vi "ParseArrayOfVariants.vi"(2 "Types":variant[](array[variant]), 6 "Type":enum16{"Indicators", "Controls"}(ring)) -> (15 "Funcdefinition":string, 16 "Description":string, 17 "FuncString":string)   [LabVIEW 2018, in "Matlab.lvclass"]
uses:
  Matlab.lvclass
  <vilib>/Utility/Data Type/NI_Data Type.lvlib
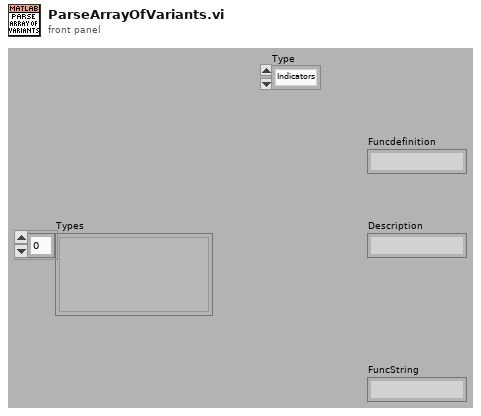
[diagram p1: front panel]
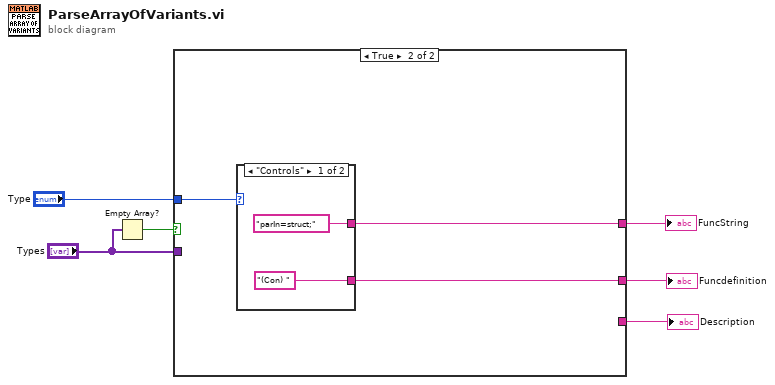
[diagram p0: block diagram]
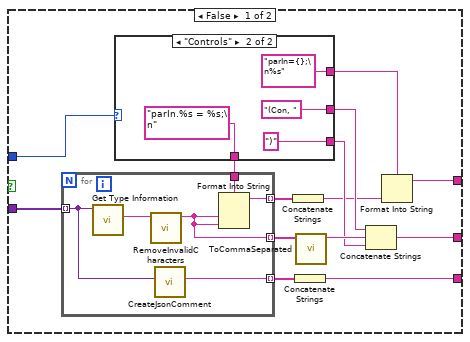
[diagram p2: hidden frame]
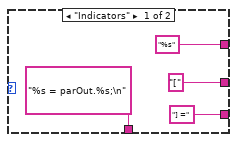
[diagram p3: hidden frame]
diagram:
  n1 = Empty Array?(array="Types") -> (empty?=w1:bool)
  n2 = case shown="True" w1 {
    tunnel: [w14 w37] -> w3
    tunnel: [w18 _] -> w2
    tunnel: [w7 w35] -> w4
    tunnel: "Types" -> [w15 _]
    tunnel: "Type" -> [w13 w36]
    frame False {
      n3 = case shown="\"Controls\"" w13 {
        tunnel: ["%s = parOut.%s;\n" ("format string") "parIn.%s = %s;\n" ("string")] -> w12
        tunnel: ["[" ("string") "(Con, " ("string")] -> w11
        tunnel: ["] =" ("string") ")" ("string")] -> w10
        tunnel: ["%s" "parIn={};\n%s"] -> w9
        frame "Indicators" {
        }
        frame "Controls" {
        }
      }
      n4 = for {
        tunnel: w15 -> [w31] mode=indexing
        tunnel: [w30] -> w19 mode=indexing
        tunnel: [w34] -> w17 mode=indexing
        tunnel: [w29] -> w16 mode=indexing
        tunnel: w12 -> [w32]
        n5 = call <vilib>:"Get Type Information.vi"("Variant"=w31) -> ("Name"=w33:string)  [unwired: 6 in, 4 out]
        n6 = call "RemoveInvalidCharacters.vi"("string in"=w33) -> ("string out"=w29:string)  [unwired: 10 in]
        n7 = call "CreateJsonComment.vi"("Variant"=w31) -> ("String"=w30:string)  [unwired: 10 in]
        n8 = Format Into String(format string=w32, w29, w29) -> (resulting string=w34:string)  [unwired: 2 in, 1 out]
      }
      n9 = Concatenate Strings(w17) -> (w8:string)
      n10 = Concatenate Strings(w19) -> (w18:string)
      n11 = call "ToCommaSeparated.vi"("Array"=w16) -> ("trimmed string"=w20:string)  [unwired: 10 in]
      n12 = Concatenate Strings(w11, w20, w10) -> (w14:string)
      n13 = Format Into String(format string=w9, w8) -> (resulting string=w7:string)  [unwired: 2 in, 1 out]
    }
    frame True {
      n14 = case shown="\"Controls\"" w36 {
        tunnel: ["(Con) " ("string") _] -> w37
        tunnel: ["parIn=struct;" _] -> w35
        frame "Controls" {
        }
        frame "Indicators" {
        }
      }
    }
  }
  "FuncString" <- w4
  "Funcdefinition" <- w3
  "Description" <- w2
